vi "2일차12vi.vi"() -> ()   [LabVIEW 2014]
panel:
  out "배열 3":dbl[](array[numeric])
  out "배열 2":dbl[](array[numeric])
  in  "배열":dbl[](array[numeric])
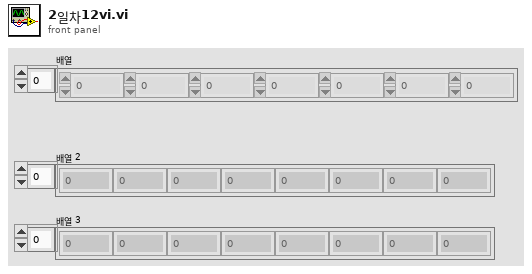
[diagram p1: front panel]
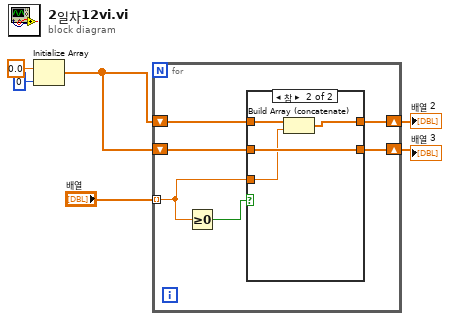
[diagram p0: block diagram]
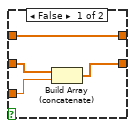
[diagram p2: hidden frame]
diagram:
  n1 = Initialize Array(0.0 ("원소"), 0 ("차원 크기")) -> (w3:dbl[])
  n2 = for {
    tunnel: "배열" -> [w7] mode=indexing
    shift-right: [w11] -> w2
    shift-left: w3 -> [w12]
    shift-right: [w9] -> w1
    shift-left: w3 -> [w10]
    n3 = Greater Or Equal To 0?(x=w7) -> (x >= 0?=w8:bool)
    n4 = case shown="참" w8 {
      tunnel: w12 -> [w16 w20]
      tunnel: [w16 w19] -> w11
      tunnel: w10 -> [w15 w18]
      tunnel: [w13 w18] -> w9
      tunnel: w7 -> [w14 w17]
      frame False {
        n5 = Build Array (concatenate)(w15, w14) -> (w13:dbl[])
      }
      frame True {
        n6 = Build Array (concatenate)(w20, w17) -> (w19:dbl[])
      }
    }
  }
  "배열 2" <- w2
  "배열 3" <- w1
